vi "ESN_Initialization.vi"(7 "ESN_AdvancedSettings":T1={"input weight matrix range (1)"=1.0, "feedweight matrix range (1)"=1.0, "output weight matrix range (0.2)"=0.2, "internal weight matrix settings"={"sparse settings (30%)"=30.0, "normalize factor (0.6)"=0.6}} {"internal weight matrix settings"."normalize factor (0.6)" min=0.0 max=1.0; "internal weight matrix settings"."sparse settings (30%)" min=0.0 max=100.0 format="%#_g%%"}, 8 "error in (no error)":errorcluster, 9 "output normalization vector":dbl[](array[numeric]), 10 "input normalization vector":dbl[](array[numeric]), 11 "UserSettingsESN":T4) -> (0 "error out":errorcluster, 3 "ESN Status":T2)   [LabVIEW 2017]
uses:
  UserSettingsESN.ctl
  ESN_Network.ctl
  <vilib>/Analysis/Matrix/Datatypes/RealMatrix.ctl
  ESN_AdvancedSettings.ctl
  <vilib>/Analysis/7linalg.llb/Eigenvalue and Vectors Output Option.ctl
  <vilib>/Analysis/7linalg.llb/Real Eigenvalues and Vectors.vi
  <vilib>/Analysis/Matrix/NI_Matrix.lvlib
  <vilib>/Analysis/NI_AALPro.lvlib
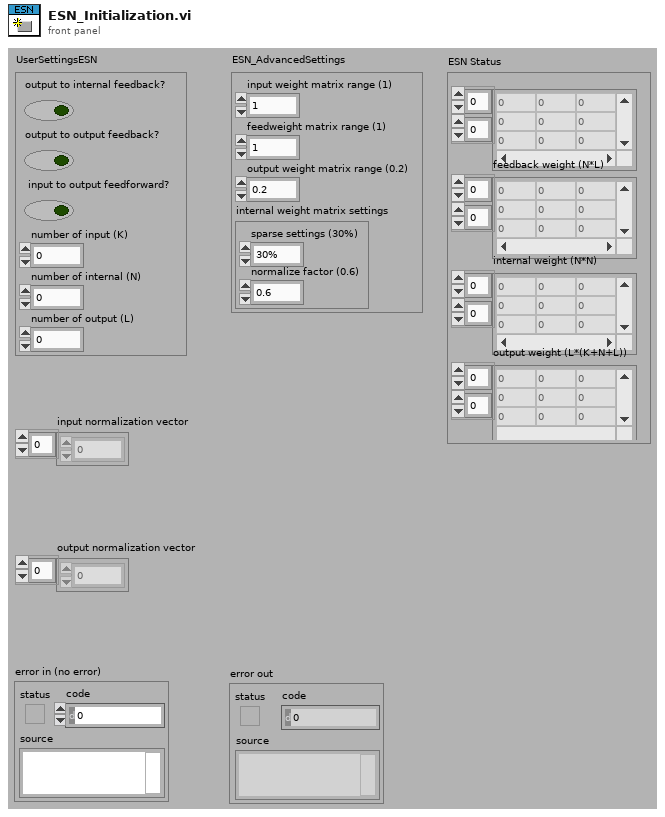
[diagram p1: front panel]
types:
  T1 = typedef "ESN_AdvancedSettings.ctl" = cluster{"input weight matrix range (1)":dbl, "feedweight matrix range (1)":dbl, "output weight matrix range (0.2)":dbl, "internal weight matrix settings":cluster{"sparse settings (30%)":dbl, "normalize factor (0.6)":dbl}}
  T2 = typedef "ESN_Network.ctl" = cluster{"output to internal feedback?":bool, "output to output feedback?":bool, "input to output feedforward?":bool, "number of input (K)":i32, "number of internal (N)":i32, "number of output (L)":i32, "input normalization vector":dbl[], "output restore vector":dbl[], "input weight (N*K)":T3, "feedback weight (N*L)":T3, "internal weight (N*N)":T3, "output weight (L*(K+N+L))":T3}
  T3 = typedef "NI_Matrix.lvlib/RealMatrix.ctl" = dbl[][]
  T4 = typedef "UserSettingsESN.ctl" = cluster{"output to internal feedback?":bool, "output to output feedback?":bool, " input to output feedforward?":bool, "number of input (K)":i32, "number of internal (N)":i32, "number of output (L)":i32}
  T5 = typedef "NI_AALPro.lvlib/Eigenvalue and Vectors Output Option.ctl" = i32
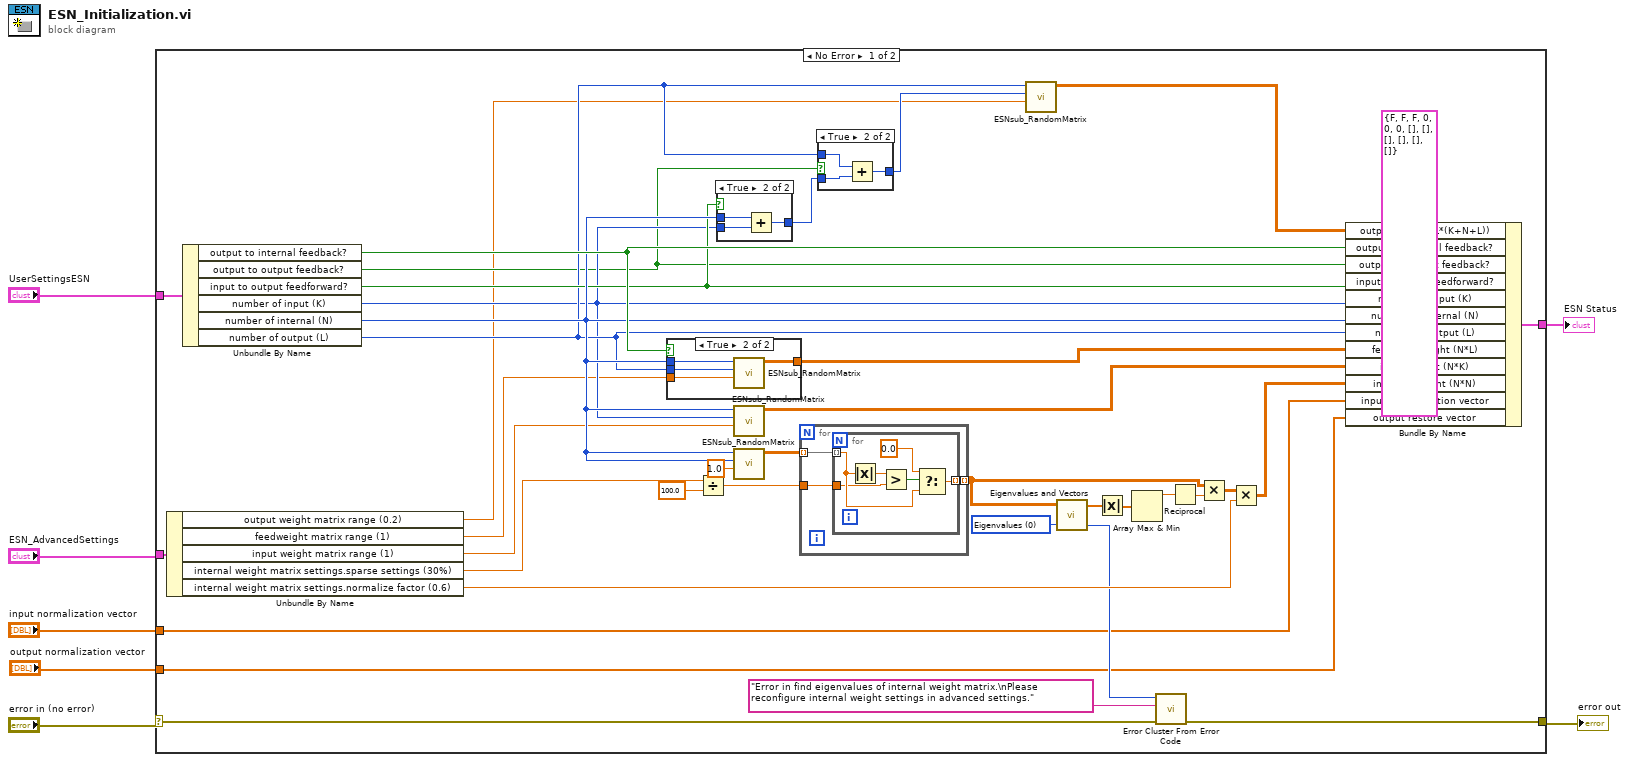
[diagram p0: block diagram]
diagram:
  n1 = case shown="No Error" "error in (no error)" {
    selector: "error in (no error)" -> [w12 w67]
    tunnel: "UserSettingsESN" -> [w45 _]
    tunnel: [w44 _] -> w6
    tunnel: "ESN_AdvancedSettings" -> [w22 _]
    tunnel: [w10 w67] -> w3
    tunnel: "input normalization vector" -> [w9 _]
    tunnel: "output normalization vector" -> [w8 _]
    frame No Error {
      w39 = T5 0 items=["Eigenvalues", "Eigenvalues & Vectors"] ("output option")
      n2 = Unbundle By Name(w22) -> ("output weight matrix range (0.2)"=w14:dbl, "feedweight matrix range (1)"=w19:dbl, "input weight matrix range (1)"=w21:dbl, "internal weight matrix settings.sparse settings (30%)"=w18:dbl, "internal weight matrix settings.normalize factor (0.6)"=w20:dbl)
      n3 = Unbundle By Name(w45) -> ("output to internal feedback?"=w33:bool, "output to output feedback?"=w23:bool, "input to output feedforward?"=w28:bool, "number of input (K)"=w25:i32, "number of internal (N)"=w29:i32, "number of output (L)"=w26:i32)
      n4 = case shown="True" w33 {
        tunnel: w29 -> [_ w66]
        tunnel: w26 -> [_ w65]
        tunnel: [_ w64] -> w41
        tunnel: w19 -> [_ w63]
        frame False {
        }
        frame True {
          n5 = call "ESNsub_RandomMatrix.vi"("Range (1)"=w63, "Column"=w65, "Row"=w66) -> ("Matrix"=w64:dbl[][])  [unwired: 8 in]
        }
      }
      n6 = Divide(x=w18, y=100.0) -> (x/y=w16:dbl)
      n7 = case shown="True" w28 {
        tunnel: w29 -> [w50 w53]
        tunnel: w25 -> [_ w52]
        tunnel: [w50 w51] -> w27
        frame False {
        }
        frame True {
          n8 = Add(x=w53, y=w52) -> (x+y=w51:i32)
        }
      }
      n9 = call "ESNsub_RandomMatrix.vi"("Range (1)"=w21, "Column"=w25, "Row"=w29) -> ("Matrix"=w42:dbl[][])  [unwired: 8 in]
      n10 = call "ESNsub_RandomMatrix.vi"("Range (1)"=1.0, "Column"=w29, "Row"=w29) -> ("Matrix"=w40:dbl[][])  [unwired: 8 in]
      n11 = for {
        tunnel: w40 -> [w56] mode=indexing
        tunnel: [w55] -> w35 mode=indexing
        tunnel: w16 -> [w54]
        n12 = for {
          tunnel: w56 -> [w59] mode=indexing
          tunnel: [w58] -> w55 mode=indexing
          tunnel: w54 -> [w57]
          n13 = Absolute Value(x=w59) -> (abs(x)=w62:dbl)
          n14 = Greater?(x=w62, y=w57) -> (0:w61:bool)
          n15 = Select(t=0.0 ("y"), s=w61, f=w59) -> (s? t:f=w58:dbl)
        }
      }
      n16 = case shown="True" w23 {
        tunnel: w27 -> [w46 w49]
        tunnel: w26 -> [_ w48]
        tunnel: [w46 w47] -> w24
        frame False {
        }
        frame True {
          n17 = Add(x=w48, y=w49) -> (x+y=w47:i32)
        }
      }
      n18 = call "ESNsub_RandomMatrix.vi"("Range (1)"=w14, "Column"=w24, "Row"=w26) -> ("Matrix"=w15:dbl[][])  [unwired: 8 in]
      n19 = call-poly <vilib>:"Eigenvalues and Vectors.vi"("output option"=w39, "Input Matrix"=w35) -> ("error"=w13:i32, "Eigenvalues"=w38:cdb[])  [unwired: 1 in, 1 out]
      n20 = Absolute Value(x=w38) -> (abs(x)=w37:dbl[])
      n21 = Array Max & Min(array=w37) -> (max value=w36:dbl)  [unwired: 3 out]
      n22 = call <vilib>:"Error Cluster From Error Code.vi"("error in (no error)"=w12, "error message (\"\")"="Error in find eigenvalues of internal weight matrix.\nPlease reconfigure internal weight settings in advanced settings." ("error message (\"\")"), "error code (0)"=w13) -> ("error out"=w10:errorcluster)  [unwired: 6 in]
      n23 = Reciprocal(x=w36) -> (1/x=w34:dbl)
      n24 = Multiply(x=w35, y=w34) -> (x*y=w32:dbl[][])
      n25 = Multiply(x=w32, y=w20) -> (x*y=w31:dbl[][])
      n26 = Bundle By Name(cluster=T2 {"output to internal feedback?"=FALSE, "output to output feedback?"=FALSE, "input to output feedforward?"=FALSE, "number of input (K)"=0, "number of internal (N)"=0, "number of output (L)"=0, "input normalization vector"=[], "output restore vector"=[], "input weight (N*K)"=[], "feedback weight (N*L)"=[], "internal weight (N*N)"=[], "output weight (L*(K+N+L))"=[]} ("ESN Status"), "output weight (L*(K+N+L))"=w15, "output to internal feedback?"=w33, "output to output feedback?"=w23, "input to output feedforward?"=w28, "number of input (K)"=w25, "number of internal (N)"=w29, "number of output (L)"=w26, "feedback weight (N*L)"=w41, "input weight (N*K)"=w42, "internal weight (N*N)"=w31, "input normalization vector"=w9, "output restore vector"=w8) -> (w44:T2)
    }
    frame Error {
    }
  }
  "ESN Status" <- w6
  "error out" <- w3
